vi "Configure Source.vi"(8 "error in (no error)":errorcluster, 10 "Source (F:Volt)":bool, 11 "E3631A in":refnum<class "E3631A.lvclass">) -> (0 "error out":errorcluster, 3 "E3631A out":refnum<class "E3631A.lvclass">)   [LabVIEW 2020, in "E3631A.lvclass"]
uses:
  E3631A.lvclass
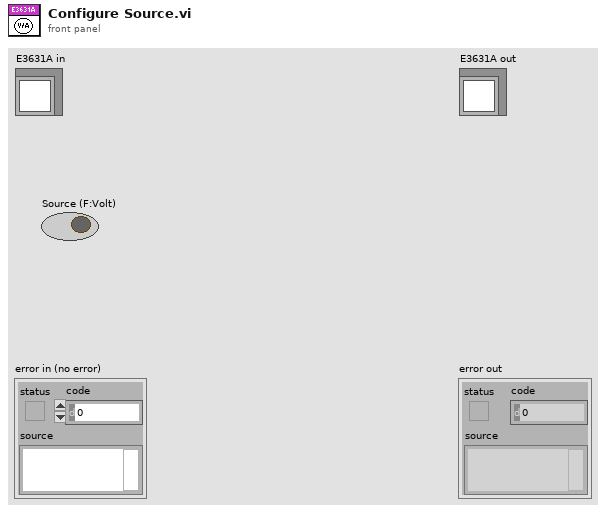
[diagram p1: front panel]
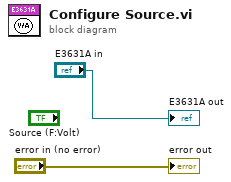
[diagram p0: block diagram]
diagram:
  "error out" <- "error in (no error)"
  "E3631A out" <- "E3631A in"
